vi "2a.vi"() -> ()   [LabVIEW 2015]
panel:
  out "Waveform Graph":dbl[][](graph)
  in  "# of samples/channel":i32=1000
  in  "Sampling rate":dbl=10000.0
  in  "physical channels":tag="Dev1/ai0:2"
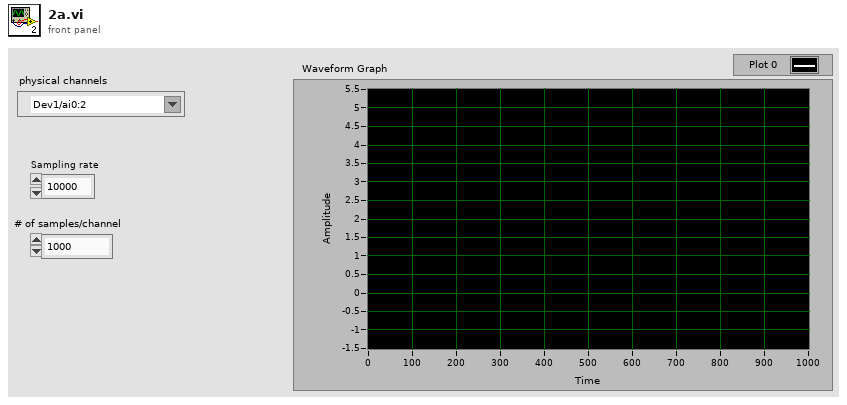
[diagram p1: front panel]
types:
  T1 = enum16{"open", "replace", "create", "open or create", "replace or create", "replace or create with confirmation"}
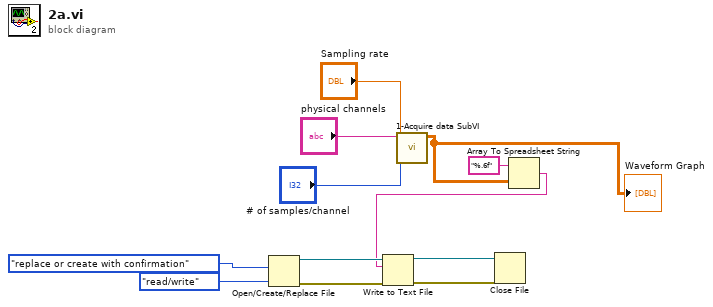
[diagram p0: block diagram]
diagram:
  n1 = Open/Create/Replace File(operation (0:open)=T1."replace or create with confirmation", access (0:read/write)=enum16{"read/write", "read-only", "write-only"}."read/write") -> (refnum out=w5:refnum<file>, error out=w7:errorcluster)  [unwired: 4 in, 1 out]
  n2 = call "1-Acquire data SubVI.vi"("# of samples/channel"="# of samples/channel", "Sampling rate"="Sampling rate", "physical channels"="physical channels") -> ("data"=w1:dbl[][])  [unwired: 8 in]
  "Waveform Graph" <- w1
  n3 = Array To Spreadsheet String(array=w1, 3:"%.6f" ("format string")) -> (spreadsheet string=w2:string)  [unwired: 1 in]
  n4 = Write to Text File(file (use dialog)=w5, text=w2, error in=w7) -> (refnum out=w4:refnum<file>, error out=w6:errorcluster)  [unwired: 1 in, 1 out]
  n5 = Close File(refnum=w4, error in=w6) -> ()  [unwired: 2 out]
